vi "PDF TESTER.vi"() -> ()   [LabVIEW 2023]
panel:
  out "return value":string[](array[string])
  out "PDF Path":string
  out "Work Order":string="XXXXX-XXX"
  out "Unit_Number":string="XXXXXXXXXXX"
  out "Path":string
  in  "System Status":string
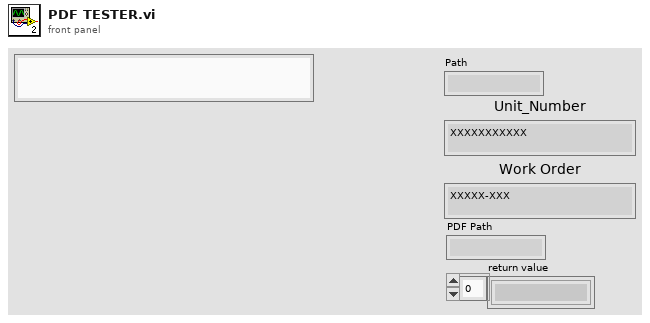
[diagram p1: front panel]
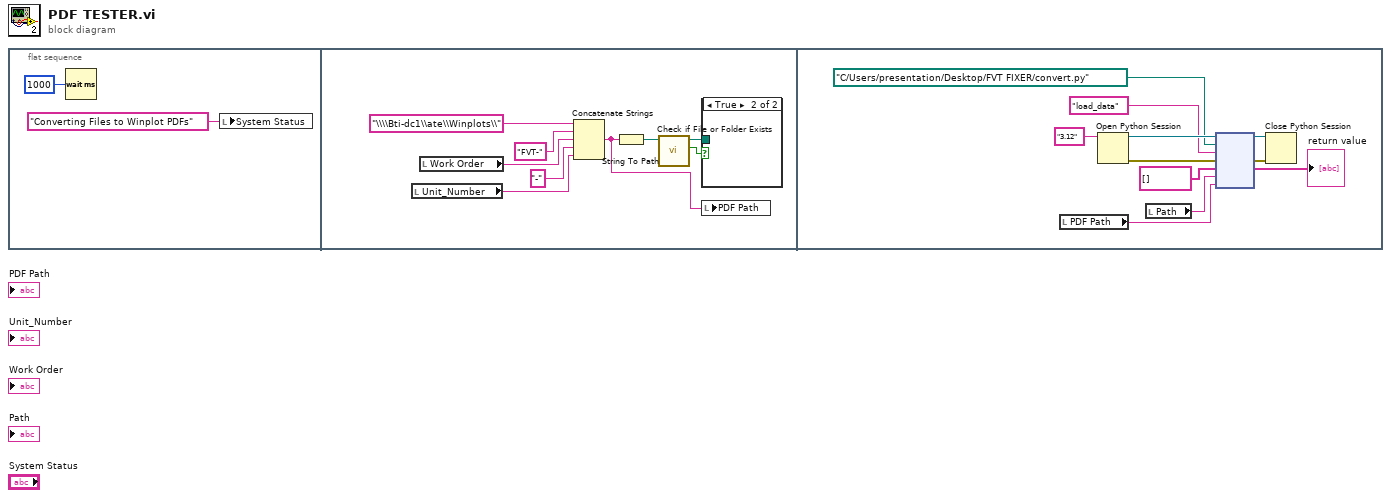
[diagram p0: block diagram]
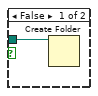
[diagram p2: hidden frame]
diagram:
  n1 = flat-sequence {
    frame #0 {
      n2 = Wait (ms)(milliseconds to wait=u32 1000) -> ()  [unwired: 1 out]
      n3 = local write "System Status"("Converting Files to Winplot PDFs") -> ()
    }
    frame #1 {
      n4 = local read "Unit_Number"() -> (w10:string)
      n5 = local read "Work Order"() -> (w11:string)
      n6 = Concatenate Strings("\\\\Bti-dc1\\ate\\Winplots\\" ("string"), "FVT-" ("string"), w11, "-" ("string"), w10) -> (w3:string)
      n7 = String To Path(string=w3) -> (path=w7:path)
      n8 = call <vilib>:"Check if File or Folder Exists.vi"("path"=w7) -> ("file or folder exists?"=w8:bool, "dup path"=w9:path)  [unwired: 8 in, 1 out]
      n9 = case shown="True" w8 {
        tunnel: w9 -> [w12 _]
        frame False {
          n10 = Create Folder(path (use dialog)=w12) -> ()  [unwired: 2 in, 3 out]
        }
        frame True {
        }
      }
      n11 = local write "PDF Path"(w3) -> ()
    }
    frame #2 {
      n12 = local read "PDF Path"() -> (w23:string)
      n13 = Open Python Session(python version="3.12" ("Python version")) -> (session out=w21:refnum<k35>, error out=w20:errorcluster)  [unwired: 2 in]
      n14 = local read "Path"() -> (w22:string)
      n15 = node(w21, path "C:/Users/presentation/Desktop/FVT FIXER/convert.py" ("module path"), "load_data" ("function name"), w20, string[] [], w22, w23) -> (w19:refnum<k35>, w18:errorcluster, →"return value":string[])  [unwired: 2 in, 2 out]
      n16 = Close Python Session(session in=w19, error in=w18) -> ()  [unwired: 1 out]
    }
  }
